vi "计时器.vi"(8 "停止":bool, 10 "开始倒计时":bool, 11 "定时时间选择":enum16{"20秒", "10秒", "6秒"}(ring)) -> (7 "?":bool, 9 "倒计时":string)   [LabVIEW 2017]
panel:
  # "计时器"
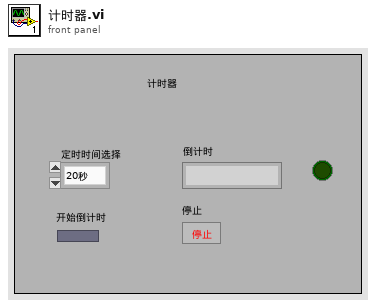
[diagram p1: front panel]
types:
  T1 = enum8{"Enabled", "Disabled", "Disabled and Grayed Out"}
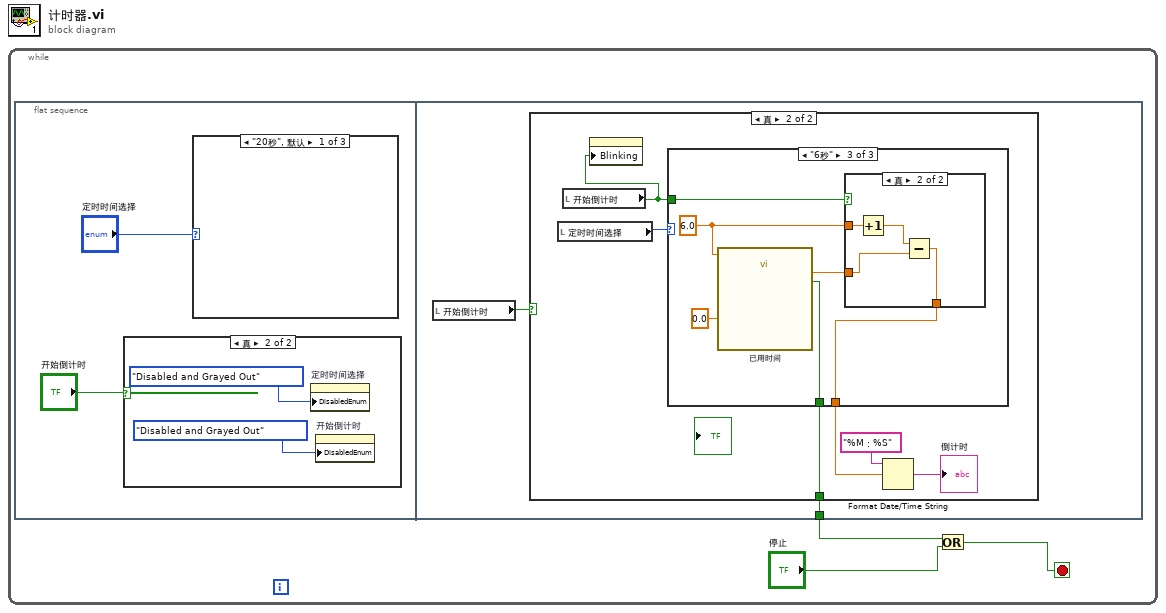
[diagram p0: block diagram]
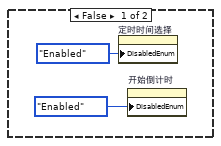
[diagram p2: hidden frame]
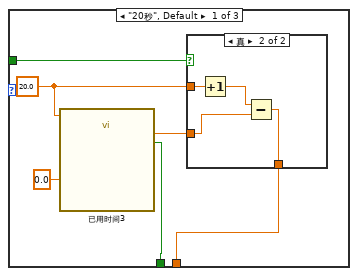
[diagram p6: hidden frame]
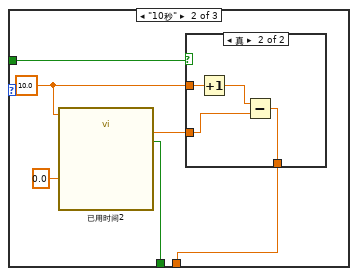
[diagram p8: hidden frame]
diagram:
  n1 = while {
    stop <- w3 stop-if-true
    n2 = flat-sequence {
      tunnel: [w10] -> w2
      frame #0 {
        n3 = case shown="真" "开始倒计时" {
          frame False {
            n4 = property on="定时时间选择" class="Enum (严格)"("DisabledEnum"=T1."Enabled" ("禁用")) -> ()  [unwired: 2 in, 2 out]
            n5 = property on="开始倒计时" class="Bool (严格)"("DisabledEnum"=T1."Enabled" ("禁用")) -> ()  [unwired: 2 in, 2 out]
          }
          frame True {
            n6 = property on="定时时间选择" class="Enum (严格)"("DisabledEnum"=T1."Disabled and Grayed Out" ("禁用")) -> ()  [unwired: 2 in, 2 out]
            n7 = property on="开始倒计时" class="Bool (严格)"("DisabledEnum"=T1."Disabled and Grayed Out" ("禁用")) -> ()  [unwired: 2 in, 2 out]
          }
        }
        n8 = case shown="\"20秒\", 默认" "定时时间选择" {
          frame "20秒", Default {
          }
          frame "10秒" {
          }
          frame "6秒" {
          }
        }
      }
      frame #1 {
        n9 = local read "开始倒计时"() -> (w11:bool)
        n10 = case shown="真" w11 {
          tunnel: [_ w13] -> w10
          frame False {
          }
          frame True {
            n11 = local read "定时时间选择"() -> (w17:enum16{"20秒", "10秒", "6秒"})
            n12 = local read "开始倒计时"() -> (w12:bool)
            n13 = property class="Bool (严格)"("Blinking"=w12) -> ()  [unwired: 2 in, 2 out]
            n14 = case shown="\"6秒\"" w17 {
              tunnel: w12 -> [w20 w31 w45]
              tunnel: [w19 w30 w41] -> w15
              tunnel: [w18 w29 w40] -> w13
              frame "20秒", Default {
                w21 = 20.0 ("Time Target (s)")
                n15 = call "已用时间3"("Time Target (s)"=w21, "Set Start Time (s)"=0.0) -> ("Elapsed Time (s)"=w23:dbl, "Time has Elapsed"=w18:bool)  [unwired: 10 in, 6 out]
                n16 = case shown="真" w20 {
                  tunnel: w23 -> [_ w26]
                  tunnel: w21 -> [w24 w28]
                  tunnel: [w24 w25] -> w19
                  frame False {
                  }
                  frame True {
                    n17 = Increment(x=w28) -> (x+1=w27:dbl)
                    n18 = Subtract(x=w27, y=w26) -> (x-y=w25:dbl)
                  }
                }
              }
              frame "10秒" {
                w32 = 10.0 ("Time Target (s)")
                n19 = call "已用时间2"("Time Target (s)"=w32, "Set Start Time (s)"=0.0) -> ("Elapsed Time (s)"=w34:dbl, "Time has Elapsed"=w29:bool)  [unwired: 10 in, 6 out]
                n20 = case shown="真" w31 {
                  tunnel: w34 -> [_ w37]
                  tunnel: w32 -> [w35 w39]
                  tunnel: [w35 w36] -> w30
                  frame False {
                  }
                  frame True {
                    n21 = Increment(x=w39) -> (x+1=w38:dbl)
                    n22 = Subtract(x=w38, y=w37) -> (x-y=w36:dbl)
                  }
                }
              }
              frame "6秒" {
                w42 = 6.0 ("Time Target (s)")
                n23 = call "已用时间"("Time Target (s)"=w42, "Set Start Time (s)"=0.0) -> ("Elapsed Time (s)"=w44:dbl, "Time has Elapsed"=w40:bool)  [unwired: 10 in, 6 out]
                n24 = case shown="真" w45 {
                  tunnel: w44 -> [_ w48]
                  tunnel: w42 -> [w46 w50]
                  tunnel: [w46 w47] -> w41
                  frame False {
                  }
                  frame True {
                    n25 = Increment(x=w50) -> (x+1=w49:dbl)
                    n26 = Subtract(x=w49, y=w48) -> (x-y=w47:dbl)
                  }
                }
              }
            }
            n27 = Format Date/Time String(time format string (%c)="%M：%S" ("时间格式字符串(%c)"), seconds (now)=w15) -> (date/time string=→"倒计时":string)  [unwired: 1 in]
          }
        }
      }
    }
    n28 = Or(x=w2, y="停止") -> (x .or. y?=w3:bool)
  }
